vi "distance.vi"(10 "target pos":dbl[](array[numeric]), 11 "obj pos":dbl[](array[numeric])) -> (2 "sqrt(x)":dbl)   [LabVIEW 2018]
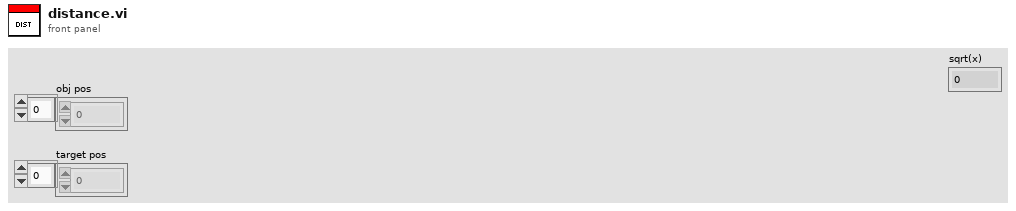
[diagram p1: front panel]
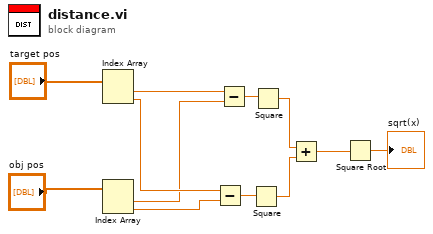
[diagram p0: block diagram]
diagram:
  n1 = Index Array(array="target pos") -> (element #1=w2:dbl, element #2=w4:dbl)  [unwired: 2 in]
  n2 = Index Array(array="obj pos") -> (element #1=w3:dbl, element #2=w5:dbl)  [unwired: 2 in]
  n3 = Subtract(x=w4, y=w5) -> (x-y=w9:dbl)
  n4 = Subtract(x=w2, y=w3) -> (x-y=w8:dbl)
  n5 = Square(x=w9) -> (x^2=w11:dbl)
  n6 = Square(x=w8) -> (x^2=w10:dbl)
  n7 = Add(x=w10, y=w11) -> (x+y=w12:dbl)
  n8 = Square Root(x=w12) -> (sqrt(x)=→"sqrt(x)":dbl)
